vi "CPP-Multiplot.vi"(0 "Plot Array":cluster{dbl[], dbl[]}[](array[cluster]) {"?" format="%.2f"; "?" format="%.2f"}, 1 "Job Directory":path) -> (2 "Saved Automatically?":bool, 3 "gnuplotScript":string, 4 "Plot data file":path)   [LabVIEW 2012]
uses:
  gnuplotScriptComponents/plotstyle.ctl
  gnuplotScriptComponents/graphPeripherals.ctl
  gnuplotScriptComponents/minAndMax.ctl
  gnuplotScriptComponents/AxisScale.ctl
  gnuplotScriptComponents/ticsAndGrids.ctl
  gnuplotScriptComponents/tics.ctl
  gnuplotScriptComponents/grids.ctl
  gnuplotScriptComponents/legendProperties.ctl
  gnuplotScriptComponents/legendAppearance.ctl
  gnuplotScriptComponents/alignment.ctl
  gnuplotScriptComponents/at.ctl
  gnuplotScriptComponents/margins.ctl
  gnuplotScriptComponents/source.ctl
  gnuplotScriptComponents/axisName.ctl
  Results_plotter_Global.vi
panel:
  in  "OpenLogfile?":bool
  in  "Show Script Editor?":bool
  in  "Tab Control":T1(tab)
  in  "ManualPlotTitles":string[](array[string])=["", "", "", "", "", "", "", "", "", "", "", "", "", "", "", ""]
  out "AutoPlotTitles":string[](array[string])
  in  "Individual Plot Titles":bool=TRUE
  in  "Page Title Pre Block":string
  in  "Page Title Post Block":string
  in  "Values to include in Page Title":i32[](listbox)
  in  "Plotstyles":T2[](array[typedef])=[{"Style"="linespoints", "Color"=16711680, "PointType"=1, "PointSize"=1.0000001, "LineWidth"=1.0, "LineType"=1}, {"Style"="linespoints", "Color"=16860, "PointType"=2, "PointSize"=1.0000001, "LineWidth"=1.0, "LineType"=1}, {"Style"="linespoints", "Color"=51228, "PointType"=3, "PointSize"=1.0, "LineWidth"=1.0, "LineType"=1}, {"Style"="linespoints", "Color"=0, "PointType"=4, "PointSize"=1.0, "LineWidth"=1.0, "LineType"=1}] caption="Style                      Colour    PointType       PointSize         Linewidth        Linestyle" {"LineType" min=1 max=6 step=1; "LineWidth" min=1 max=6 step=1; "PointSize" min=0 step=0.1}
  out "No of Graph Slots Available":i32
  out "No of Series supplied":i32
  in  "Title Offset (characters)":cluster{"horizontal":dbl, "vertical":dbl}
  in  "Each Graph contains:":T3=enum."Series"
  in  "Rows from:":T3=enum."Until done"
  in  "Columns from:":T3=enum."Selector 1"
  in  "Margins":T4={"Top"=2.0, "Bottom"=2.0, "Left"=2.0, "Right"=2.0}
  in  "Height (in)":dbl=7.0 min=0.5 step=0.5 format="%.1f"
  in  "Width (in)":dbl=10.0 min=0.5 step=0.5 format="%.1f"
  in  "nRows":u8=3 min=1
  in  "nCols":u8=3 min=1
  in  "ScaleAdjust":dbl=0.9 min=0.1 max=2.0 step=0.1
  in  "X axis label":enum32{"Autolabel", "Manual Label"}(tab)
  out "X or theta label":string
  in  "X or theta label Manual":string
  in  "LegendProperties":T5={"Appearance"={"layout"="", "text-sample order"="", "key order"="", "surroundingBox"=""}, "Alignment"={"Horizontal"="", "Vertical"=""}, "Location"="auto", "\"At\" location"={"XcoordSys"="", "YcoordSys"="", "Xvalue"=0.0, "Yvalue"=0.0}}
  in  "Y/R tics And Grids":T9={"tics"={"Auto"=TRUE, "ticMin"=-10.0, "ticStep"=1.0, "ticMax"=10.0, "minorDivsPerMajor"=2, "Mirror tics"=TRUE}, "Grids"={"Gridlines"=enum."Major grid", "Zeroaxis"=enum."No zero axis"}}
  in  "X/Theta tics And Grids":T9={"tics"={"Auto"=TRUE, "ticMin"=-10.0, "ticStep"=1.0, "ticMax"=10.0, "minorDivsPerMajor"=2, "Mirror tics"=TRUE}, "Grids"={"Gridlines"=enum."Major grid", "Zeroaxis"=enum."No zero axis"}}
  in  "PlotType":enum32{"XY", "Polar"}(tab)
  in  "yAxisBounds":T12={"Min"={"Auto"=TRUE, "Value"=0.0}, "Max"={"Auto"=TRUE, "Value"=0.0}}
  in  "Additional XYgnuplot":string
  in  "xAxisBounds":T12={"Min"={"Auto"=TRUE, "Value"=0.0}, "Max"={"Auto"=TRUE, "Value"=0.0}}
  in  "Angle Units":bool=TRUE
  in  "AngleMode":string(combo)="Compass"
  in  "wrapGapsUpTo:":dbl=30.0 step=0.1
  in  "Additional Polar gnuplot":string
  in  "rAxisBounds":T12={"Min"={"Auto"=FALSE, "Value"=0.0}, "Max"={"Auto"=FALSE, "Value"=1.5}}
  in  "Y axis label":enum32{"Autolabel", "Manual Label"}(tab)
  out "Y or R label":string
  in  "Y or R label Manual 2":string
  in  "Edge Axis Labels only":bool=TRUE
  in  "GraphPeripherals":T14[][](array[typedef])
  out "PlotCommand":string
  in  "Filename Max length":i32=255
  out "Path":path
  out "Final Title":string
  out "AuditTrail":string[](array[string])
  out "Plot Legends":string[](array[string])
  out "Desired Legends":string[][](array[string])
  # "Overall Page Title"
  # "Plot Styles"
  # "There are as many graphs as there are titles (from Selector 2)...."
  # "And each graph contains plots from Selector 1..."
  # "Rows/ Columns/ Series from: controls not wired- just a thought for explicit control of what goes where...?"
  # "X/theta"
  # "Y/r"
  # "Shows the numbered line colours and point styles available"
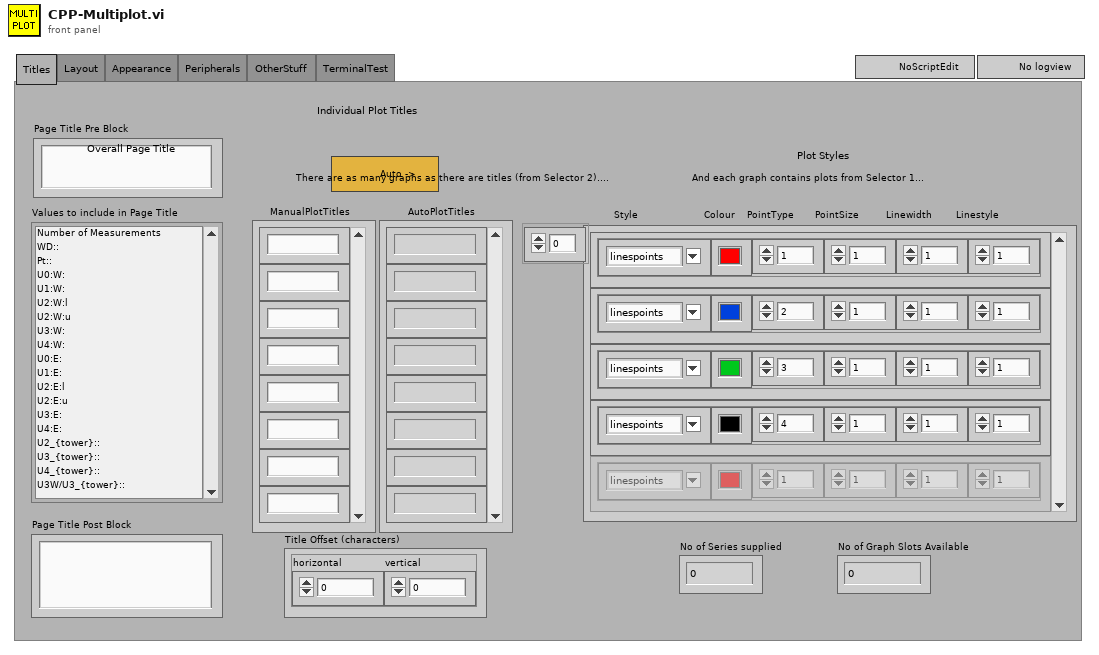
[diagram p1: front panel]
types:
  T1 = enum32{"Titles", "Layout", "Appearance", "Peripherals", "OtherStuff ", "TerminalTest"}
  T2 = typedef "plotstyle.ctl" = cluster{"Style":string, "Color":u32, "PointType":i32, "PointSize":sgl, "LineWidth":sgl, "LineType":u8}
  T3 = typedef "source.ctl" = enum16{"Specified:", "Selector 1", "Selector 2", "Until done", "Series"}
  T4 = typedef "margins.ctl" = cluster{"Top":dbl, "Bottom":dbl, "Left":dbl, "Right":dbl}
  T5 = typedef "legendProperties.ctl" = cluster{"Appearance":T6, "Alignment":T7, "Location":string, "\"At\" location":T8}
  T6 = typedef "legendAppearance.ctl" = cluster{"layout":string, "text-sample order":string, "key order":string, "surroundingBox":string}
  T7 = typedef "alignment.ctl" = cluster{"Horizontal":string, "Vertical":string}
  T8 = typedef "at.ctl" = cluster{"XcoordSys":string, "YcoordSys":string, "Xvalue":dbl, "Yvalue":dbl}
  T9 = typedef "ticsAndGrids.ctl" = cluster{"tics":T10, "Grids":T11}
  T10 = typedef "tics.ctl" = cluster{"Auto":bool, "ticMin":dbl, "ticStep":dbl, "ticMax":dbl, "minorDivsPerMajor":i32, "Mirror tics":bool}
  T11 = typedef "grids.ctl" = cluster{"Gridlines":enum16{"No grids", "Major grid", "Minor grid", "Major and Minor"}, "Zeroaxis":enum16{"No zero axis", "Show zero axis"}}
  T12 = typedef "minAndMax.ctl" = cluster{"Min":T13, "Max":T13}
  T13 = typedef "AxisScale.ctl" = cluster{"Auto":bool, "Value":dbl}
  T14 = typedef "graphPeripherals.ctl" = cluster{"title":bool, "key":bool, "Xtic":bool, "Ytic":bool, "Xlab":bool, "Ylab":bool}
  T15 = typedef "axisName.ctl" = string
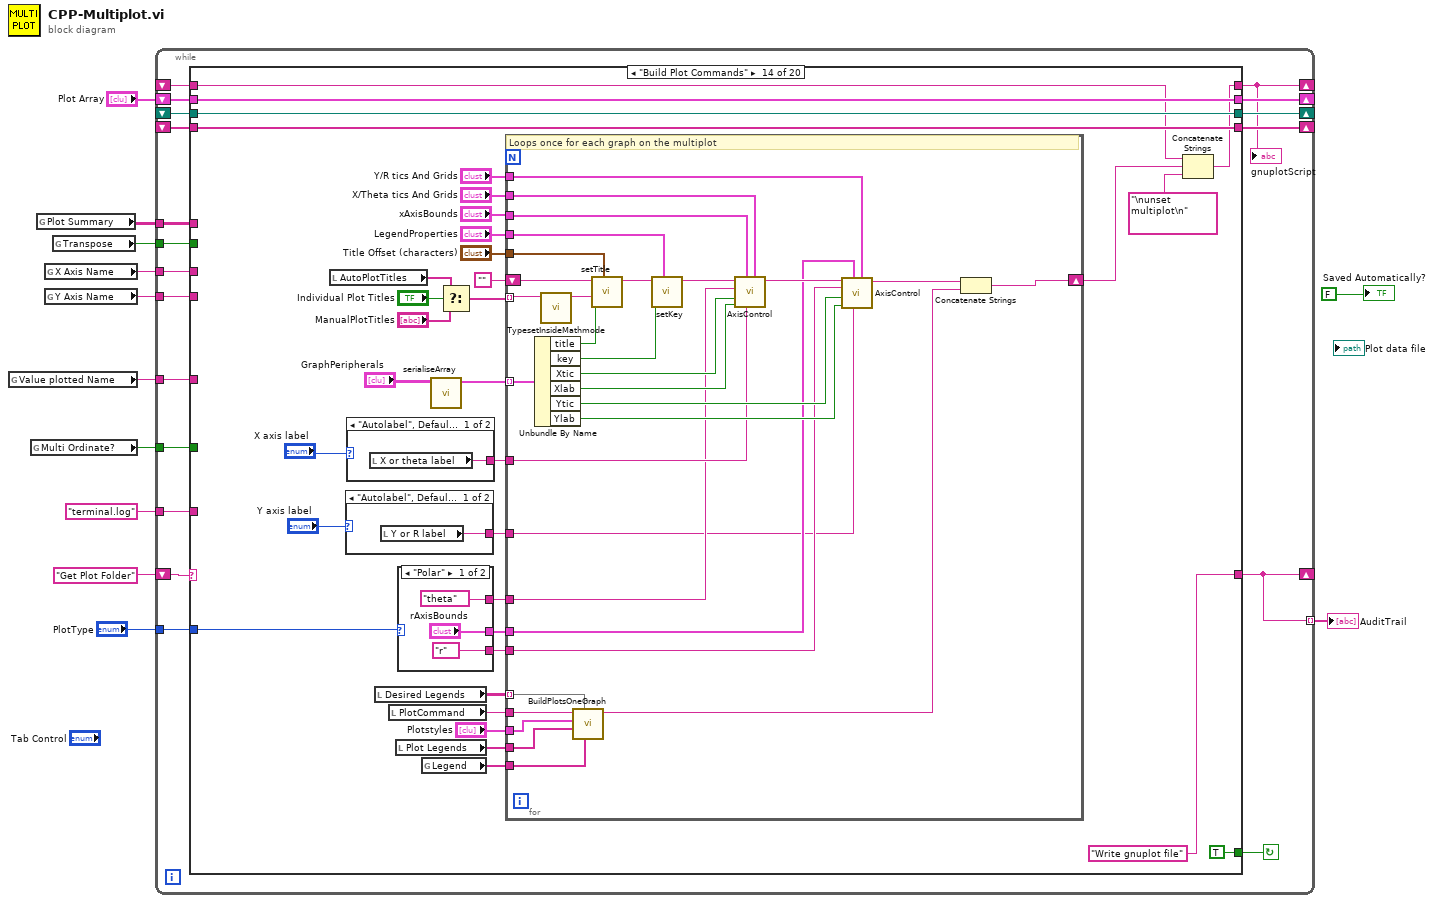
[diagram p0: block diagram]
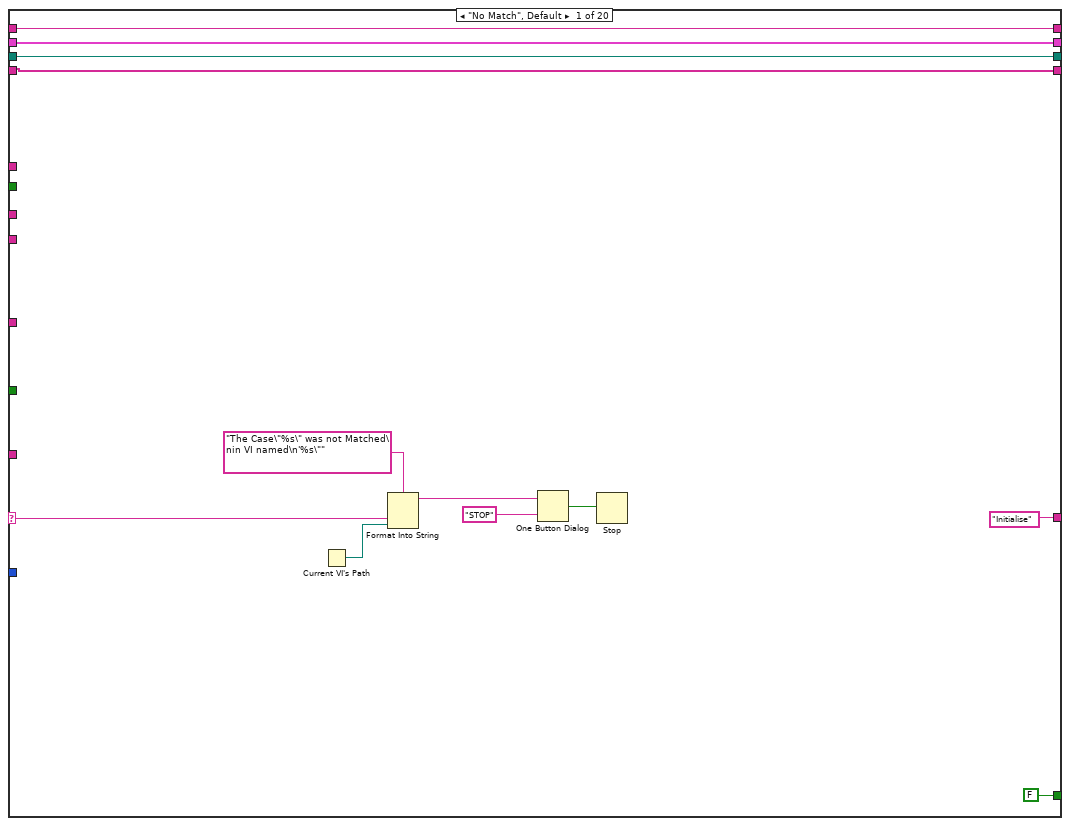
[diagram p2: hidden frame]
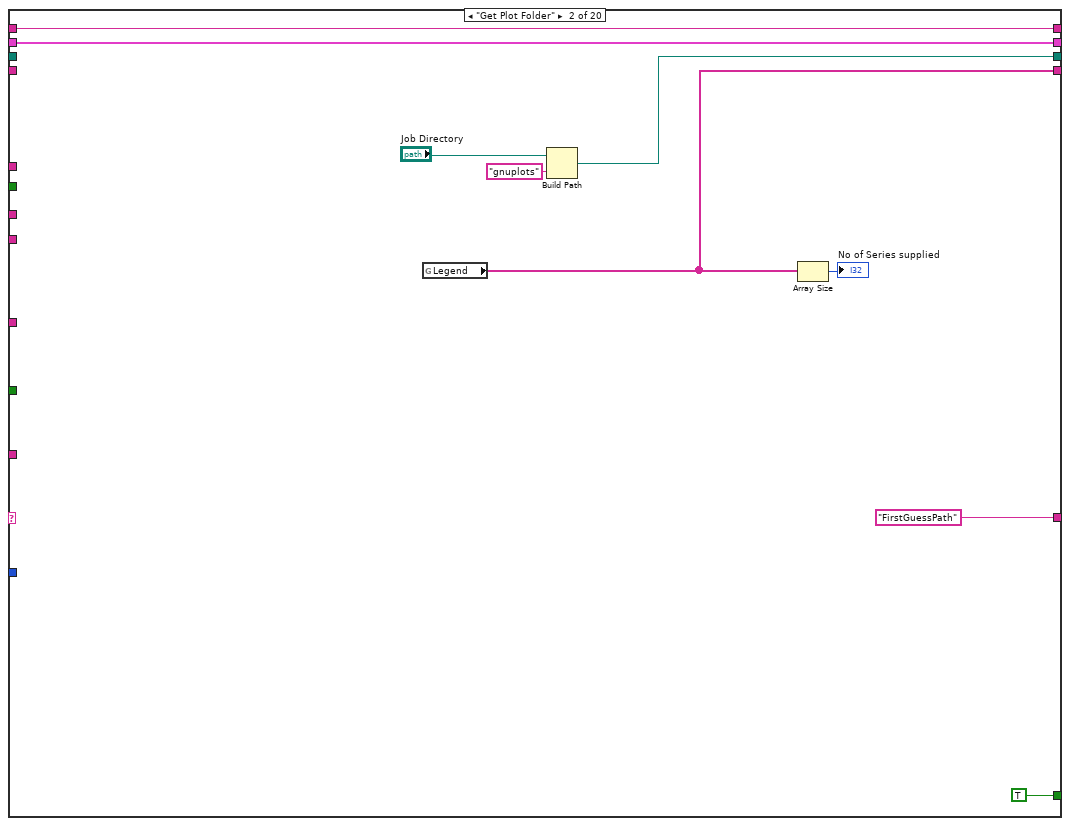
[diagram p3: hidden frame]
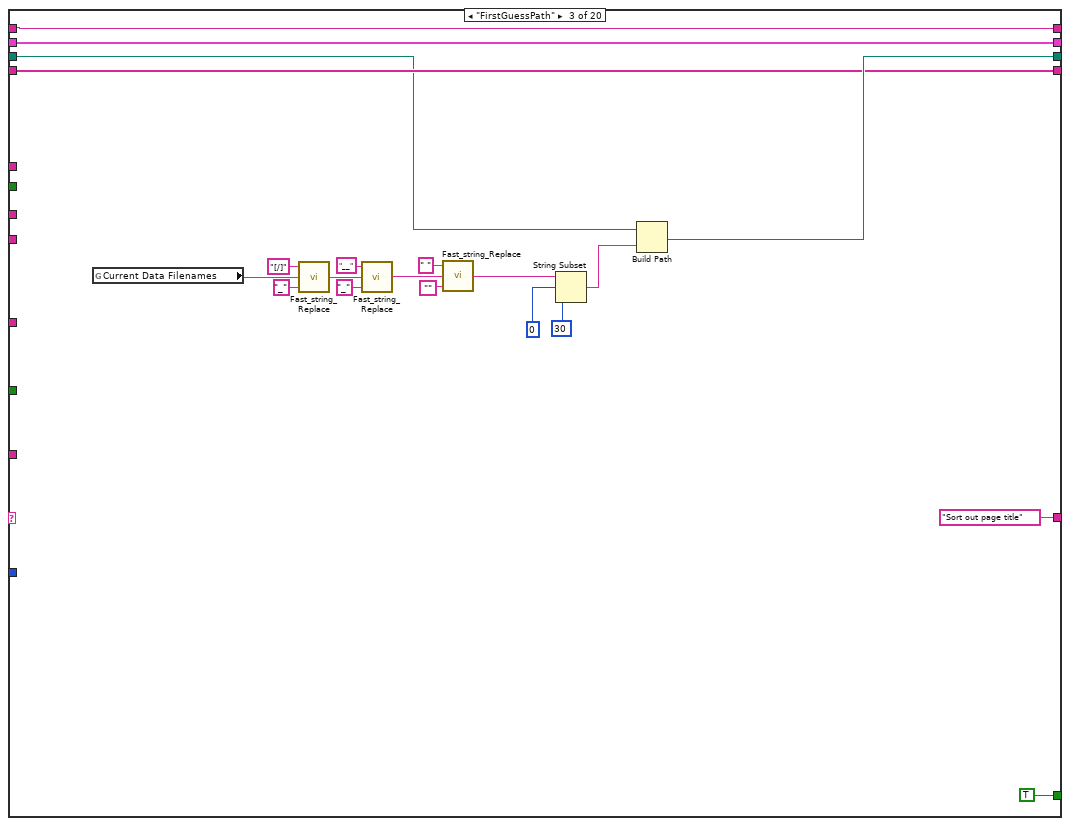
[diagram p4: hidden frame]
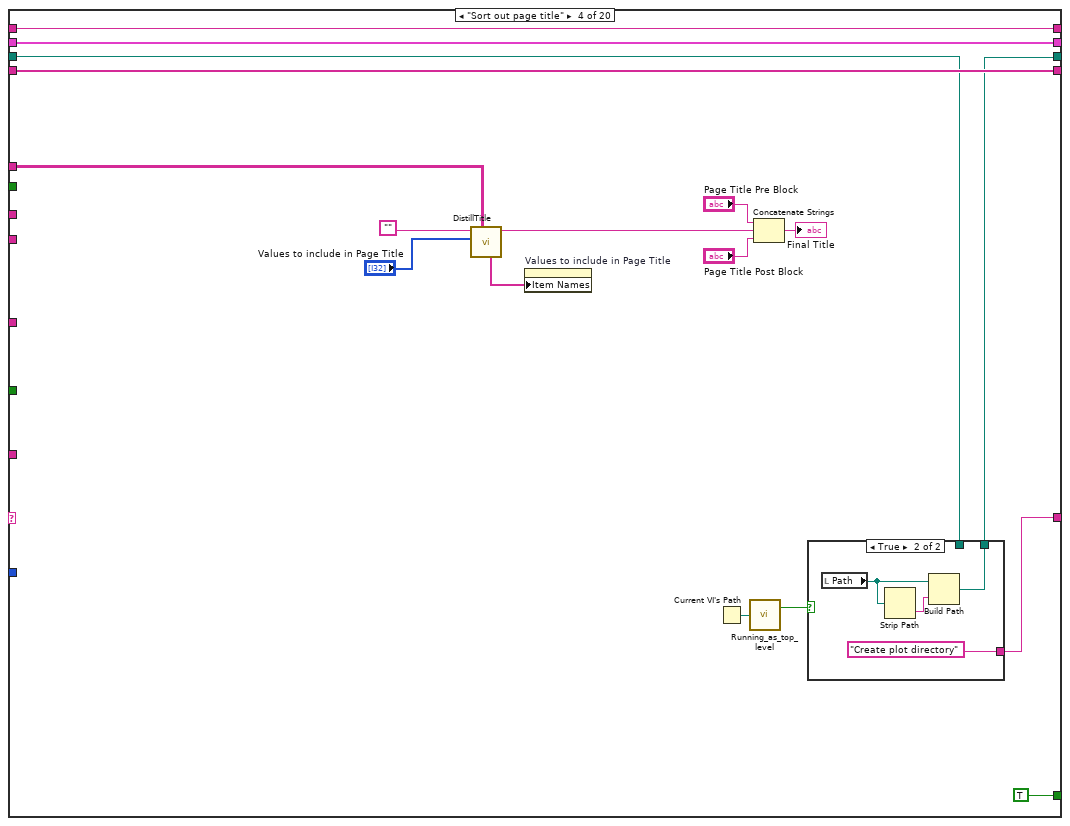
[diagram p5: hidden frame]
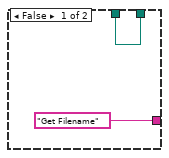
[diagram p6: hidden frame]
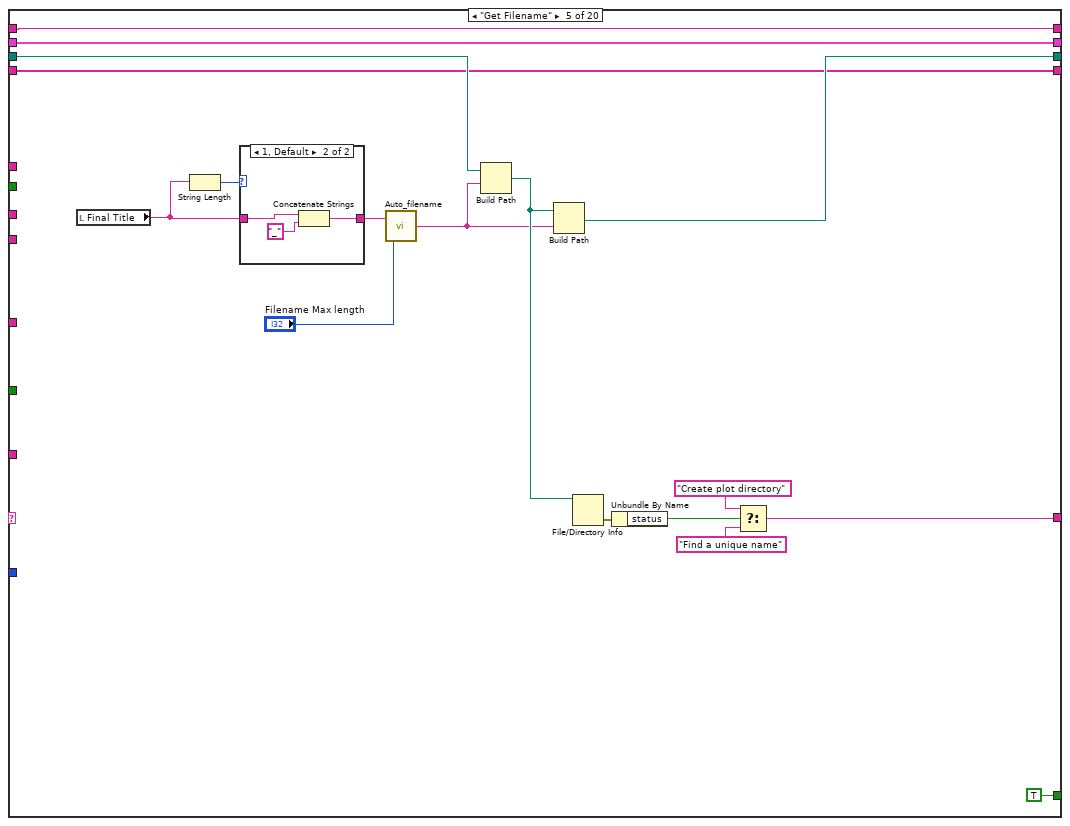
[diagram p7: hidden frame]
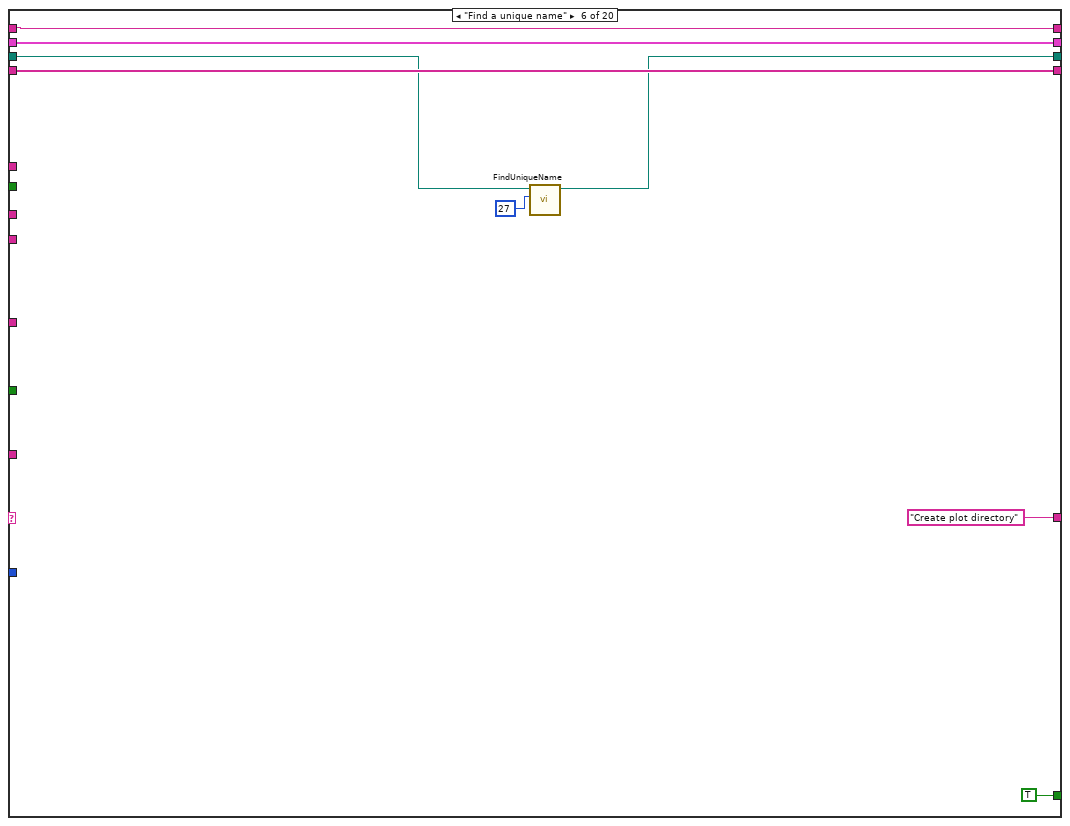
[diagram p9: hidden frame]
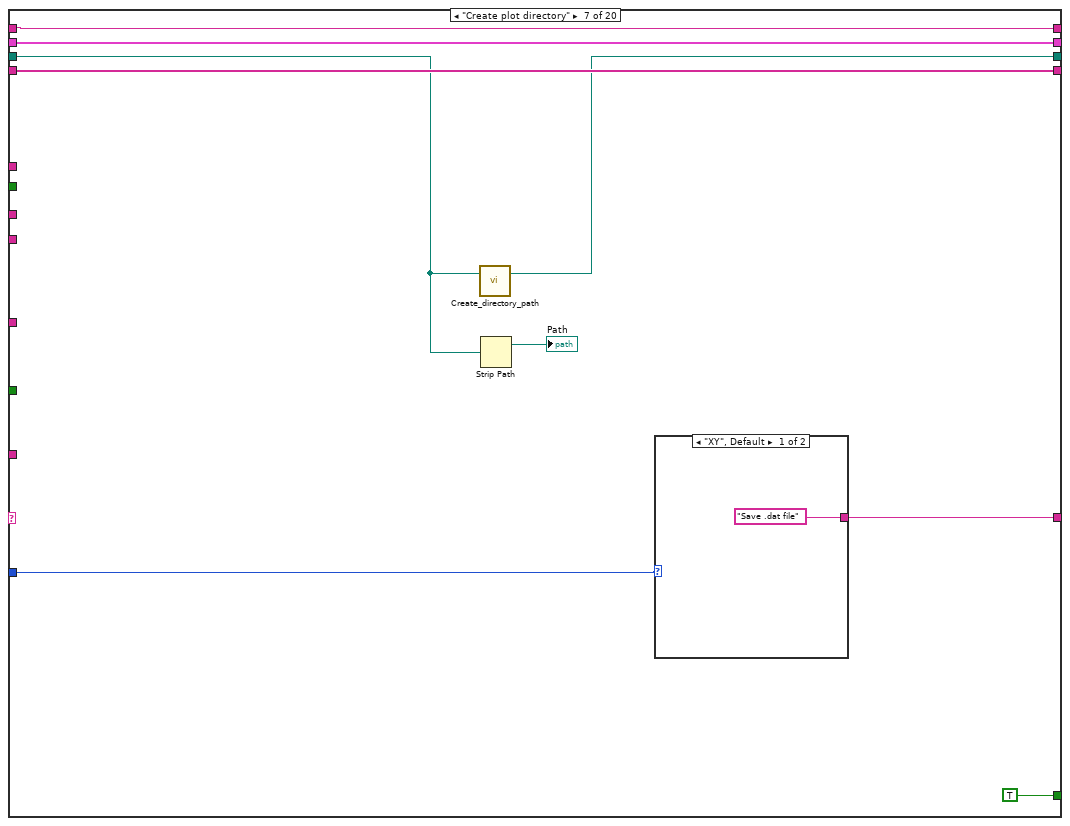
[diagram p10: hidden frame]
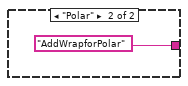
[diagram p11: hidden frame]
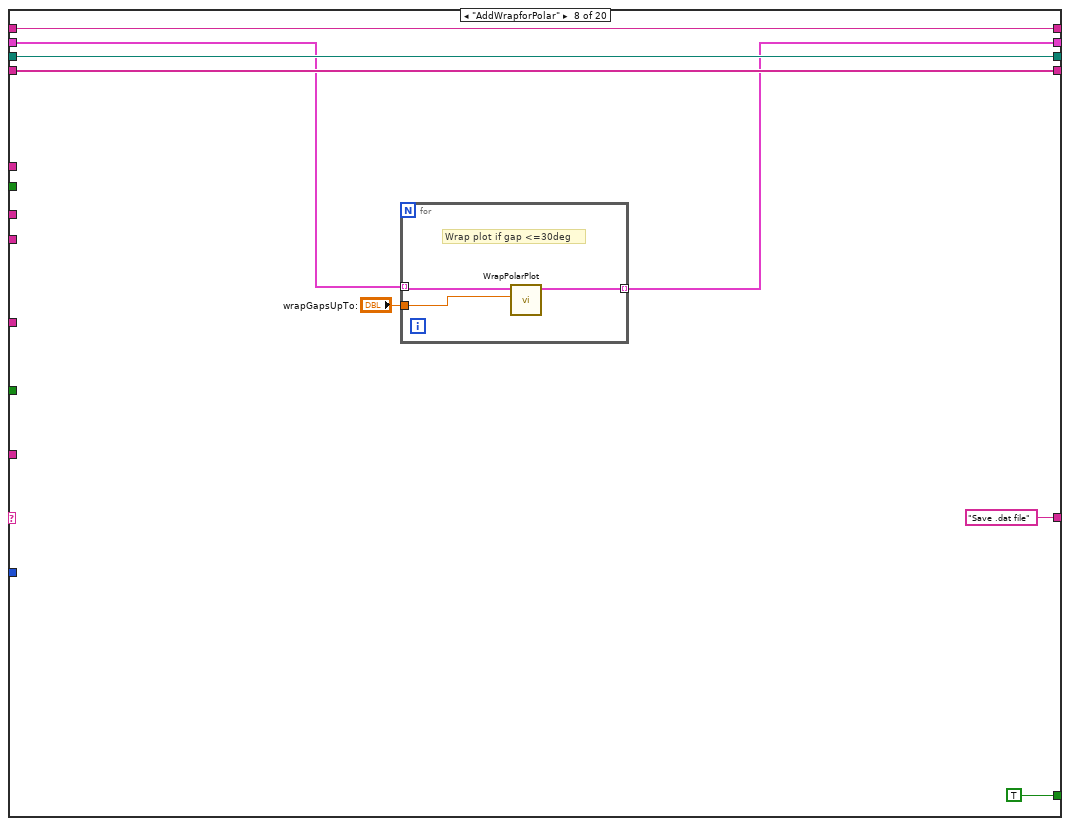
[diagram p12: hidden frame]
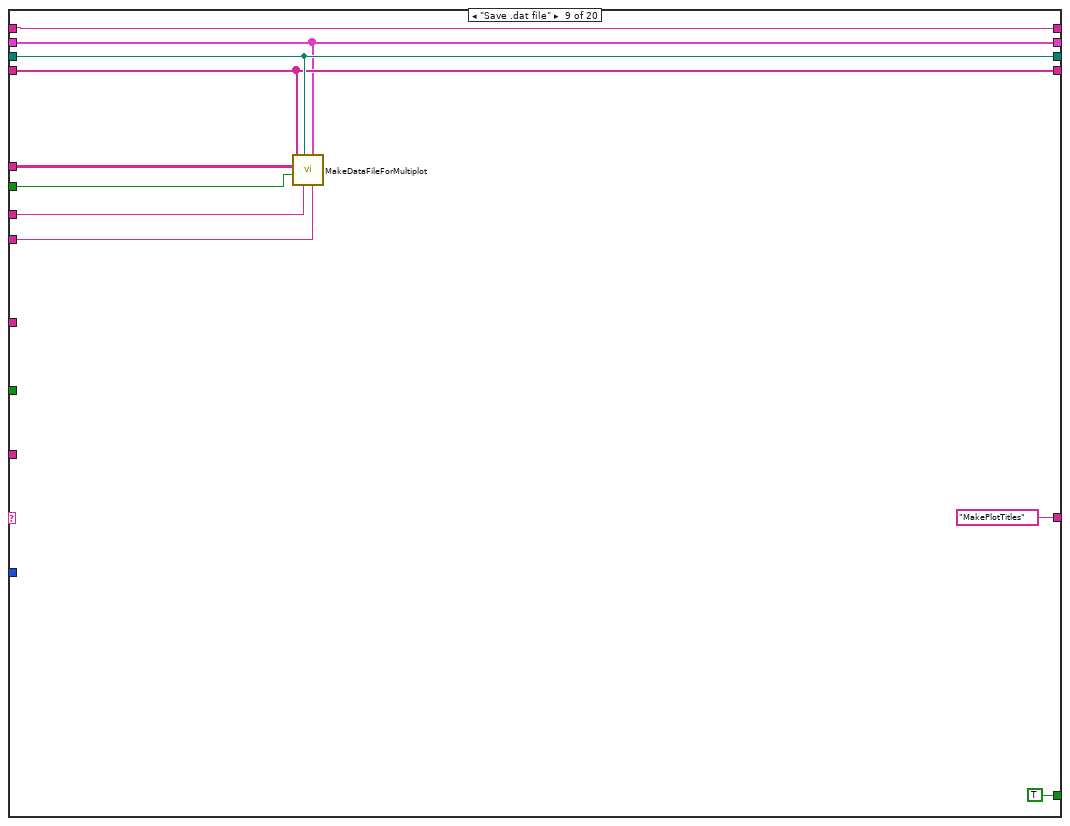
[diagram p13: hidden frame]
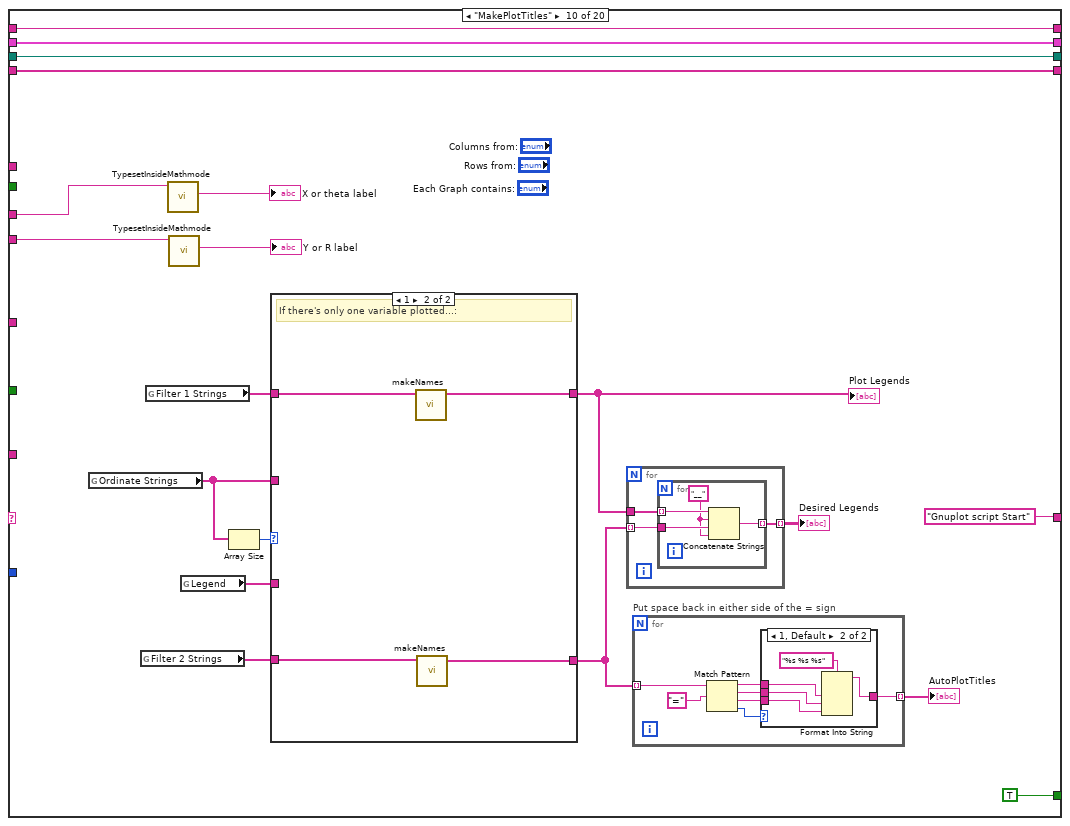
[diagram p14: hidden frame]
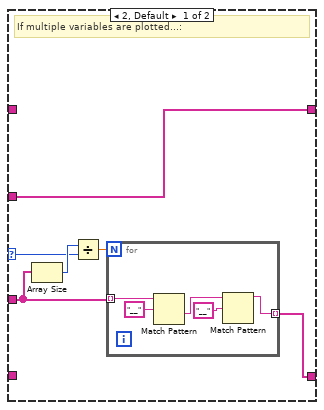
[diagram p16: hidden frame]
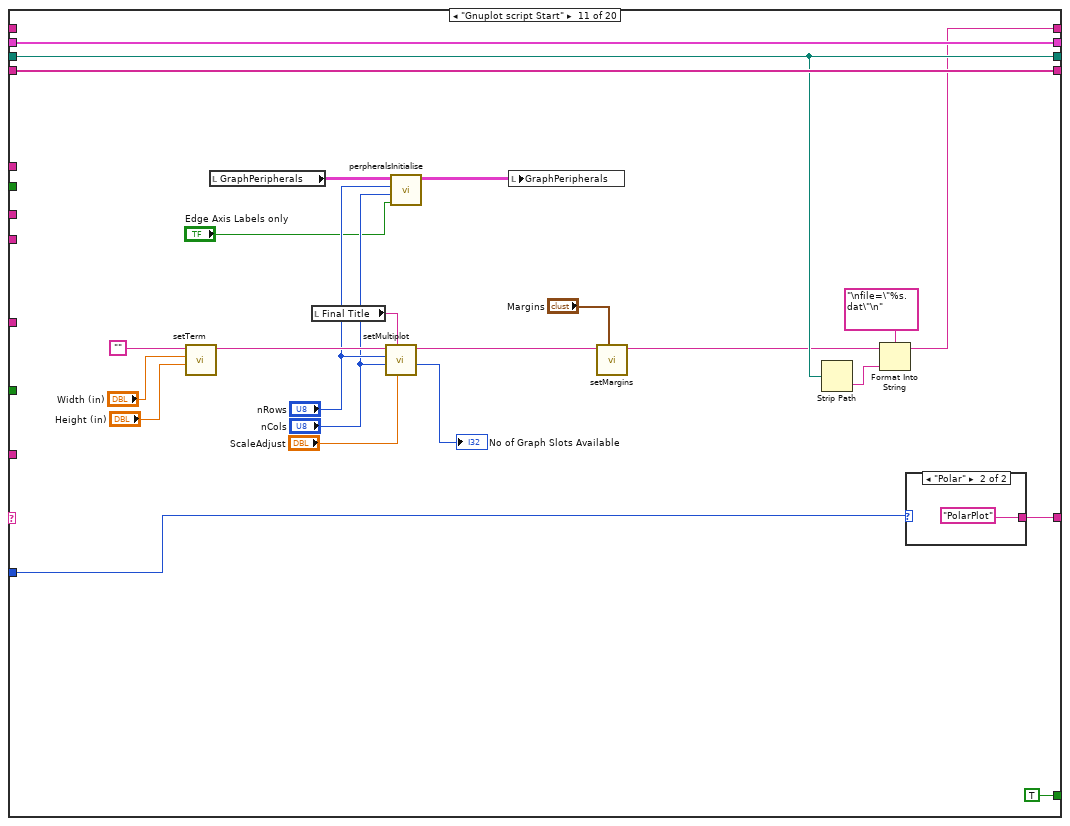
[diagram p17: hidden frame]
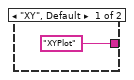
[diagram p18: hidden frame]
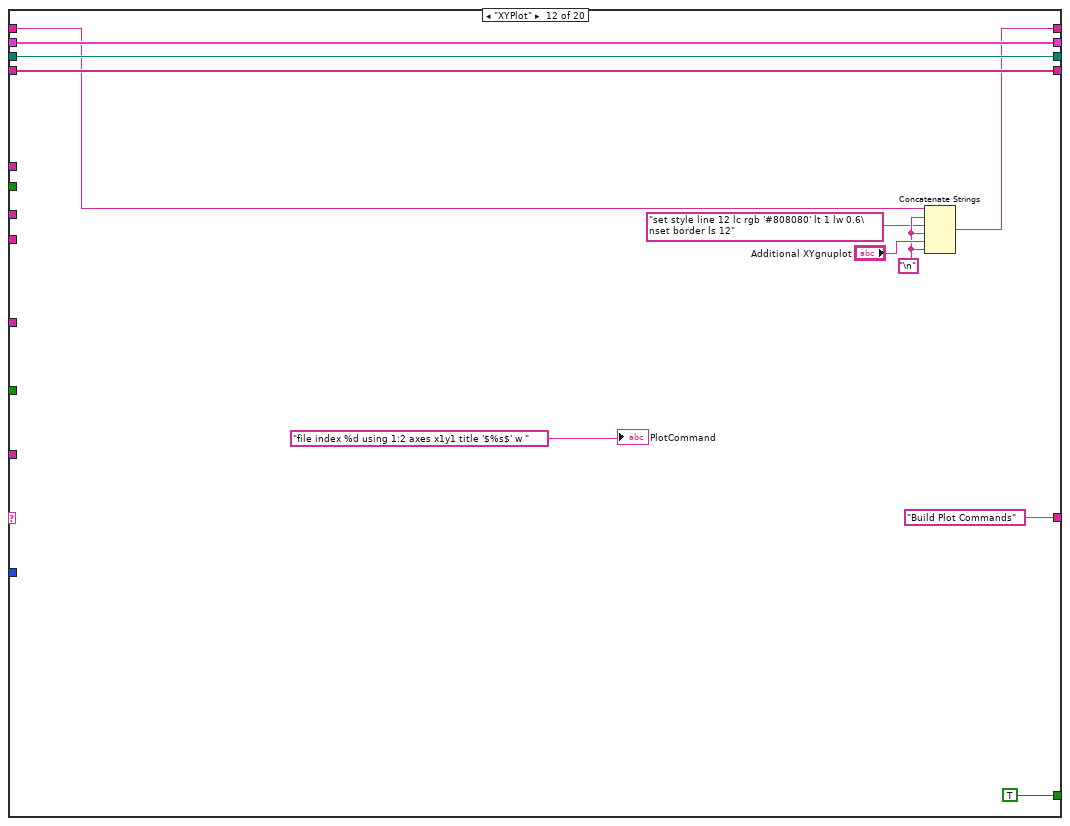
[diagram p19: hidden frame]
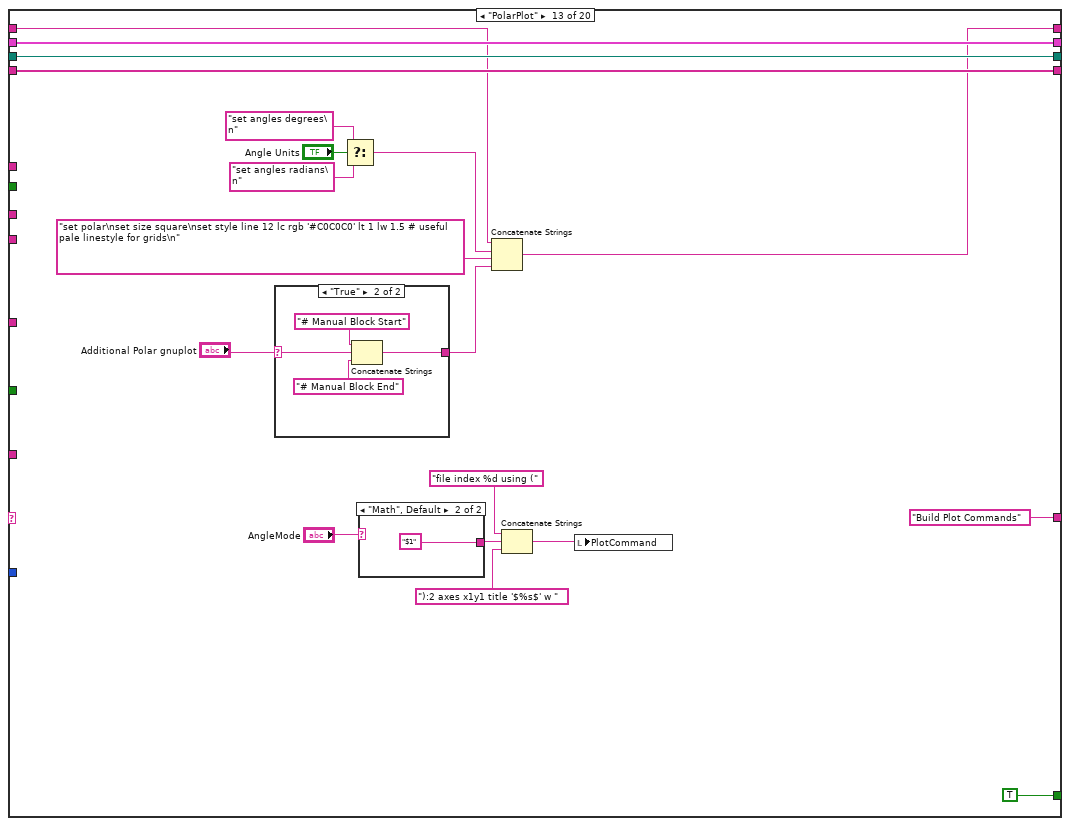
[diagram p20: hidden frame]
diagram:
  n1 = global read "Results_plotter_Global.vi" "Value plotted Name"() -> (w8:string)
  n2 = global read "Results_plotter_Global.vi" "Multi Ordinate?"() -> (w3:bool)
  n3 = global read "Results_plotter_Global.vi" "Plot Summary"() -> (w11:string[][])
  n4 = global read "Results_plotter_Global.vi" "X Axis Name"() -> (w10:string)
  n5 = global read "Results_plotter_Global.vi" "Y Axis Name"() -> (w9:string)
  n6 = global read "Results_plotter_Global.vi" "Transpose"() -> (w4:bool)
  n7 = while {
    shift-left: "Get Plot Folder" -> [w30]
    shift-right: [w14] -> _
    tunnel: w11 -> [w29]
    shift-right: [w28] -> _
    shift-left: _ -> [w27]
    tunnel: w10 -> [w26]
    tunnel: w9 -> [w25]
    tunnel: w8 -> [w24]
    shift-right: [w22] -> _
    shift-left: "Plot Array" -> [w23]
    shift-right: [w15] -> _
    shift-left: _ -> [w21]
    shift-right: [w20] -> _
    shift-left: _ -> [w19]
    tunnel: "terminal.log" -> [w18]
    tunnel: w4 -> [w17]
    tunnel: w3 -> [w16]
    tunnel: [w14] -> w2 mode=indexing
    tunnel: "PlotType" -> [w13]
    stop <- w31 continue-if-true
    n8 = case shown="\"Build Plot Commands\"" w30 {
      selector: w30 -> [w32 _ _ _ _ _ _ _ _ _ _ _ _ _ _ _ _ _ _ _]
      tunnel: [FALSE TRUE TRUE ("Top Level") TRUE ("Top Level") TRUE ("Top Level") TRUE ("Top Level") TRUE TRUE ("Top Level") TRUE ("Top Level") TRUE ("Top Level") TRUE ("Top Level") TRUE ("Top Level") TRUE ("Top Level") TRUE ("Top Level") TRUE ("Top Level") TRUE ("Top Level") TRUE ("Top Level") FALSE ("Top Level") TRUE ("Top Level") FALSE ("Top Level")] -> w31
      tunnel: ["Initialise" "FirstGuessPath" "Sort out page title" w81 w110 "Create plot directory" w125 "Save .dat file" "MakePlotTitles" "Gnuplot script Start" w231 "Build Plot Commands" "Build Plot Commands" "Write gnuplot file" ("t") "Execute shell script" ("t") "Has pdf been generated?" ("t") w371 "End" "End" ("t") "End" ("t")] -> w14
      tunnel: w29 -> [_ _ _ w75 _ _ _ _ w154 _ _ _ _ _ _ _ _ _ _ _]
      tunnel: [w36 w50 w72 w83 w111 w117 w130 w142 w155 w175 w222 w247 w265 w306 w353 w361 w375 w380 w390 w401] -> w28
      tunnel: w27 -> [w36 _ w68 w82 w107 w118 w129 w142 w155 w175 w222 w247 w265 w306 w353 w361 w375 w380 w390 w401]
      tunnel: w26 -> [_ _ _ _ _ _ _ _ w153 w168 _ _ _ _ _ _ _ _ _ _]
      tunnel: w25 -> [_ _ _ _ _ _ _ _ w152 w167 _ _ _ _ _ _ _ _ _ _]
      tunnel: w24 -> [_ _ _ _ _ _ _ _ _ _ _ _ _ _ _ _ _ _ _ _]
      tunnel: w23 -> [w35 w46 w71 w89 w109 w121 w133 w138 w149 w174 w234 w246 w266 w307 w359 w366 w378 w385 w395 w400]
      tunnel: [w35 w46 w71 w89 w109 w121 w133 w137 w149 w174 w234 w246 w266 w307 w359 w366 w378 w385 w395 w400] -> w22
      tunnel: w21 -> [w34 w49 w70 w87 w108 w120 w132 w143 w156 w173 _ w237 w260 w298 w349 w364 w376 w383 w393 w399]
      tunnel: [w34 w49 w70 w87 w108 w120 w132 w143 w156 w173 w219 w241 w261 w304 w349 w364 w376 w383 w393 w399] -> w15
      tunnel: [w33 w45 w69 w88 w106 w119 w131 w141 w151 w172 w233 w245 w264 w305 w354 w365 w377 w384 w394 w398] -> w20
      tunnel: w19 -> [w33 _ w69 w88 w106 w119 w131 w141 w151 w172 w233 w245 w264 w305 w354 w365 w377 w384 w394 w398]
      tunnel: w18 -> [_ _ _ _ _ _ _ _ _ _ _ _ _ _ _ w360 _ _ w388 _]
      tunnel: w17 -> [_ _ _ _ _ _ _ _ w150 _ _ _ _ _ _ _ _ _ _ _]
      tunnel: w16 -> [_ _ _ _ _ _ _ _ _ _ _ _ _ _ _ _ _ _ _ _]
      tunnel: w13 -> [_ _ _ _ _ _ w126 _ _ _ w218 _ _ w282 _ _ _ _ _ _]
      frame "No Match", Default {
        n9 = Current VI's Path() -> (path=w38:path)
        n10 = Format Into String(format string="The Case\"%s\" was not Matched\nin VI named\n'%s\"" ("Format String"), w32, w38) -> (resulting string=w41:string)  [unwired: 2 in, 1 out]
        n11 = One Button Dialog(message=w41, button name ("OK")="STOP") -> (true=w39:bool)
        n12 = Stop(stop? (T)=w39) -> ()
      }
      frame "Get Plot Folder" {
        n13 = global read "Results_plotter_Global.vi" "Legend"() -> (w45:string[])
        n14 = Build Path(base path="Job Directory", name or relative path="gnuplots") -> (appended path=w50:path)
        n15 = Array Size(array=w45) -> (size(s)=→"No of Series supplied":i32)
      }
      frame "FirstGuessPath" {
        n16 = global read "Results_plotter_Global.vi" "Current Data Filenames"() -> (w57:string)
        n17 = call "Fast_string_Replace.vi"("Replace match with:"="_", "Input String"=w57, "regular expression"="[/]") -> ("Output String"=w61:string)  [unwired: 2 out]
        n18 = call "Fast_string_Replace.vi"("Replace match with:"="_", "Input String"=w61, "regular expression"="__") -> ("Output String"=w58:string)  [unwired: 2 out]
        n19 = call "Fast_string_Replace.vi"("Replace match with:"="", "Input String"=w58, "regular expression"=" ") -> ("Output String"=w56:string)  [unwired: 2 out]
        n20 = String Subset(string=w56, offset (0)=0, length (rest)=30 ("length (rest)")) -> (substring=w55:string)
        n21 = Build Path(base path=w68, name or relative path=w55) -> (appended path=w72:path)
      }
      frame "Sort out page title" {
        n22 = call "DistillTitle.vi"("Plot Summary in"=w75, "Indices to include in Page Title"="Values to include in Page Title", "String in"="") -> ("String out"=w80:string, "AvailableVariables"=w73:string[])  [unwired: 7 in]
        n23 = property on="Values to include in Page Title" class="LstBox (strict)"("Item Names"=w73) -> ()  [unwired: 2 in, 2 out]
        n24 = Current VI's Path() -> (path=w86:path)
        n25 = call "Running_as_top_level.vi"("Vi path name"=w86) -> ("Top Level"=w84:bool)  [unwired: 1 out]
        n26 = Concatenate Strings("Page Title Pre Block", w80, "Page Title Post Block") -> (→"Final Title":string)
        n27 = case shown="True" w84 {
          tunnel: [w91 w94] -> w83
          tunnel: w82 -> [w91 _]
          tunnel: ["Get Filename" ("t") "Create plot directory"] -> w81
          frame False {
          }
          frame True {
            n28 = local read "Path"() -> (w93:path)
            n29 = Strip Path(path=w93) -> (name=w92:string)  [unwired: 1 out]
            n30 = Build Path(base path=w93, name or relative path=w92) -> (appended path=w94:path)
          }
        }
      }
      frame "Get Filename" {
        n31 = local read "Final Title"() -> (w96:string)
        n32 = String Length(string=w96) -> (length=w98:i32)
        n33 = case shown="1, Default" w98 {
          tunnel: [w113 w114] -> w97
          tunnel: w96 -> [w113 w116]
          frame 0 {
          }
          frame 1, Default {
            n34 = Concatenate Strings(w116, "_") -> (w114:string)
          }
        }
        n35 = call "Auto_filename.vi"("Filename Max length"="Filename Max length", "Prefix"=w97) -> ("Filename"=w100:string)
        n36 = Build Path(base path=w107, name or relative path=w100) -> (appended path=w104:path)
        n37 = Build Path(base path=w104, name or relative path=w100) -> (appended path=w111:path)
        n38 = File/Directory Info(path=w104) -> (error out=w105:errorcluster)  [unwired: 1 in, 6 out]
        n39 = Unbundle By Name(w105) -> ("status"=w103:bool)
        n40 = Select(t="Create plot directory", s=w103, f="Find a unique name") -> (s? t:f=w110:string)
      }
      frame "Find a unique name" {
        n41 = call "FindUniqueName.vi"("Max Length"=27, "PathIn"=w118) -> ("UniquedPath"=w117:path)  [unwired: 9 in]
      }
      frame "Create plot directory" {
        n42 = call "Create_directory_path.vi"("Path name"=w129) -> ("Path name Out"=w130:path)  [unwired: 1 in, 1 out]
        n43 = Strip Path(path=w129) -> (stripped path=→"Path":path)  [unwired: 1 out]
        n44 = case shown="\"XY\", Default" w126 {
          tunnel: ["Save .dat file" "AddWrapforPolar"] -> w125
          frame "XY", Default {
          }
          frame "Polar" {
          }
        }
      }
      frame "AddWrapforPolar" {
        n45 = for {
          tunnel: w138 -> [w146] mode=indexing
          tunnel: [w145] -> w137 mode=indexing
          tunnel: "wrapGapsUpTo:" -> [w144]
          # "Wrap plot if gap <=30deg"
          n46 = call "WrapPolarPlot.vi"("maxWrap"=w144, "thetaRin"=w146) -> ("thetaRout"=w145:cluster{"Angle":dbl[], "Radius":dbl[]})  [unwired: 9 in]
        }
      }
      frame "Save .dat file" {
        n47 = call "MakeDataFileForMultiplot.vi"("Y Axis Name"=w152, "Plot Array"=w149, "X Axis Name"=w153, "Path"=w155, "Transpose"=w150, "Plot Summary"=w154, "Legend"=w151) -> ()  [unwired: 5 in]
      }
      frame "MakePlotTitles" {
        n48 = global read "Results_plotter_Global.vi" "Ordinate Strings"() -> (w166:string[])
        n49 = global read "Results_plotter_Global.vi" "Filter 2 Strings"() -> (w163:string[])
        n50 = global read "Results_plotter_Global.vi" "Filter 1 Strings"() -> (w164:string[])
        n51 = call "TypesetInsideMathmode.vi"("DirtyString"=w168) -> ("Mathmode String"=→"X or theta label":string)  [unwired: 9 in, 1 out]
        n52 = call "TypesetInsideMathmode.vi"("DirtyString"=w167) -> ("Mathmode String"=→"Y or R label":string)  [unwired: 9 in, 1 out]
        n53 = global read "Results_plotter_Global.vi" "Legend"() -> (w170:string[])
        n54 = Array Size(array=w166) -> (size(s)=w159:i32)
        n55 = case shown="1" w159 {
          selector: w159 -> [w196 _]
          tunnel: w170 -> [w199 _]
          tunnel: [w201 w208] -> w162
          tunnel: [w200 w210] -> w160
          tunnel: w166 -> [w200 _]
          tunnel: w164 -> [_ w209]
          tunnel: w163 -> [_ w207]
          frame 2, Default {
            # "If multiple variables are plotted...:"
            n56 = Array Size(array=w199) -> (size(s)=w198:i32)
            n57 = Divide(x=w198, y=w196) -> (x/y=w197:dbl)
            n58 = for {
              N: w197 -> [_]
              tunnel: w199 -> [w205] mode=indexing
              tunnel: [w202] -> w201 mode=indexing
              n59 = Match Pattern(string=w205, regular expression="__") -> (after substring=w203:string)  [unwired: 1 in, 3 out]
              n60 = Match Pattern(string=w203, regular expression="__") -> (before substring=w202:string)  [unwired: 1 in, 3 out]
            }
          }
          frame 1 {
            # "If there's only one variable plotted...:"
            n61 = call "makeNames.vi"("Strings"=w209) -> ("Names"=w210:string[])  [unwired: 10 in]
            n62 = call "makeNames.vi"("Strings"=w207) -> ("Names"=w208:string[])  [unwired: 10 in]
          }
        }
        "Plot Legends" <- w160
        n63 = for {
          tunnel: w160 -> [w191]
          tunnel: w162 -> [w190] mode=indexing
          tunnel: [w189] -> w165 mode=indexing
          n64 = for {
            tunnel: w191 -> [w195] mode=indexing
            tunnel: w190 -> [w194]
            tunnel: [w193] -> w189 mode=indexing
            w192 = "__" ("string")
            n65 = Concatenate Strings(w195, w192, w194, w192) -> (w193:string)
          }
        }
        "Desired Legends" <- w165
        n66 = for "Put space back in either side of the = sign" {
          tunnel: w162 -> [w182] mode=indexing
          tunnel: [w177] -> w161 mode=indexing
          n67 = Match Pattern(string=w182, regular expression="=") -> (before substring=w180:string, match substring=w179:string, after substring=w178:string, offset past match=w176:i32)  [unwired: 1 in]
          n68 = case shown="1, Default" w176 {
            tunnel: w180 -> [w183 w188]
            tunnel: w179 -> [_ w187]
            tunnel: w178 -> [_ w186]
            tunnel: [w183 w185] -> w177
            frame -1 {
            }
            frame 1, Default {
              n69 = Format Into String(format string="%s %s %s", w188, w187, w186) -> (resulting string=w185:string)  [unwired: 2 in, 1 out]
            }
          }
        }
        "AutoPlotTitles" <- w161
      }
      frame "Gnuplot script Start" {
        n70 = call "setTerm.vi"("Height (in)"="Height (in)", "Width (in)"="Width (in)", "String in"="") -> ("String out"=w227:string)  [unwired: 7 in, 1 out]
        n71 = local read "GraphPeripherals"() -> (w213:T14[][])
        n72 = local read "Final Title"() -> (w225:string)
        n73 = call "setMultiplot.vi"("ScaleAdjust"="ScaleAdjust", "OverallTitle"=w225, "Cols"="nCols", "Rows"="nRows", "String in"=w227) -> ("nGraphs"=→"No of Graph Slots Available":i32, "String out"=w226:string)  [unwired: 4 in, 1 out]
        n74 = call "perpheralsInitialise.vi"("Edge Axis Labels only"="Edge Axis Labels only", "Cols"="nCols", "Rows"="nRows", "GraphPeripheralsIn"=w213) -> ("GraphPeripheralsOut"=w214:T14[][])  [unwired: 7 in]
        n75 = local write "GraphPeripherals"(w214) -> ()
        n76 = call "setMargins.vi"("Margins"="Margins", "String in"=w226) -> ("String out"=w217:string)  [unwired: 8 in, 1 out]
        n77 = Strip Path(path=w222) -> (name=w221:string)  [unwired: 1 out]
        n78 = Format Into String(format string="\nfile=\"%s.dat\"\n" ("string"), initial string=w217, w221) -> (resulting string=w219:string)  [unwired: 1 in, 1 out]
        n79 = case shown="\"Polar\"" w218 {
          tunnel: ["XYPlot" "PolarPlot"] -> w231
          frame "XY", Default {
          }
          frame "Polar" {
          }
        }
      }
      frame "XYPlot" {
        w240 = "\n"
        n80 = Concatenate Strings(w237, w240, "set style line 12 lc rgb '#808080' lt 1 lw 0.6\nset border ls 12" ("input 2"), w240, "Additional XYgnuplot", w240) -> (w241:string)
        "PlotCommand" <- "file index %d using 1:2 axes x1y1 title '$%s$' w " ("format string")
      }
      frame "PolarPlot" {
        n81 = case shown="\"True\"" "Additional Polar gnuplot" {
          selector: "Additional Polar gnuplot" -> [w267 w271]
          tunnel: [w267 w270] -> w248
          frame "\u0000", Default {
          }
          frame "True" {
            n82 = Concatenate Strings("# Manual Block Start" ("string"), w271, "# Manual Block End" ("string")) -> (w270:string)
          }
        }
        n83 = Select(t="set angles degrees\n", s="Angle Units", f="set angles radians\n") -> (s? t:f=w250:string)
        n84 = case shown="\"Math\", Default" "AngleMode" {
          tunnel: ["90-$1" ("format string") "$1" ("format string")] -> w255
          frame "Compass" {
          }
          frame "Math", Default {
          }
        }
        n85 = Concatenate Strings(w260, w250, "set polar\nset size square\nset style line 12 lc rgb '#C0C0C0' lt 1 lw 1.5 # useful pale linestyle for grids\n", w248) -> (w261:string)
        n86 = Concatenate Strings("file index %d using (" ("format string"), w255, "):2 axes x1y1 title '$%s$' w " ("format string")) -> (w254:string)
        n87 = local write "PlotCommand"(w254) -> ()
      }
      frame "Build Plot Commands" {
        n88 = local read "AutoPlotTitles"() -> (w296:string[])
        n89 = case shown="\"Autolabel\", Default" "Y axis label" {
          tunnel: [w308 "Y or R label Manual 2"] -> w277
          frame "Autolabel", Default {
            n90 = local read "Y or R label"() -> (w308:string)
          }
          frame "Manual Label" {
          }
        }
        n91 = case shown="\"Autolabel\", Default" "X axis label" {
          tunnel: [w316 "X or theta label Manual"] -> w283
          frame "Autolabel", Default {
            n92 = local read "X or theta label"() -> (w316:string)
          }
          frame "Manual Label" {
          }
        }
        n93 = local read "Desired Legends"() -> (w290:string[][])
        n94 = local read "PlotCommand"() -> (w285:string)
        n95 = local read "Plot Legends"() -> (w291:string[])
        n96 = case shown="\"Polar\"" w282 {
          tunnel: [T15 "theta" ("Axis") T15 "x" ("Axis")] -> w280
          tunnel: [T15 "r" ("Axis") T15 "y" ("Axis")] -> w279
          tunnel: ["rAxisBounds" "yAxisBounds"] -> w281
          frame "Polar" {
          }
          frame Default {
          }
        }
        n97 = global read "Results_plotter_Global.vi" "Legend"() -> (w289:string[])
        n98 = call "serialiseArray.vi"("GraphPeripherals"="GraphPeripherals") -> ("output array"=w292:T14[])  [unwired: 10 in]
        n99 = Select(t=w296, s="Individual Plot Titles", f="ManualPlotTitles") -> (s? t:f=w294:string[])
        n100 = for {
          shift-right: [w346] -> w299
          shift-left: "" -> [w344]
          tunnel: w291 -> [w347]
          tunnel: "Plotstyles" -> [w348]
          tunnel: w294 -> [w330] mode=indexing
          tunnel: w292 -> [w343] mode=indexing
          tunnel: w290 -> [w333] mode=indexing
          tunnel: w289 -> [w332]
          tunnel: "LegendProperties" -> [w329]
          tunnel: "Title Offset (characters)" -> [w327]
          tunnel: w285 -> [w326]
          tunnel: w283 -> [w325]
          tunnel: w281 -> [w324]
          tunnel: w280 -> [w323]
          tunnel: w279 -> [w322]
          tunnel: w277 -> [w321]
          tunnel: "Y/R tics And Grids" -> [w320]
          tunnel: "X/Theta tics And Grids" -> [w319]
          tunnel: "xAxisBounds" -> [w318]
          # "Loops once for each graph on the multiplot"
          n101 = Unbundle By Name(w343) -> ("title"=w342:bool, "key"=w340:bool, "Xtic"=w337:bool, "Xlab"=w336:bool, "Ytic"=w335:bool, "Ylab"=w334:bool)
          n102 = call "TypesetInsideMathmode.vi"("DirtyString"=w330) -> ("De-dollared String"=w331:string)  [unwired: 9 in, 1 out]
          n103 = call "BuildPlotsOneGraph.vi"("Legend"=w332, "Desired Legends"=w333, "Plot Legends"=w347, "Plotstyles"=w348, "PlotCommand"=w326) -> ("String out"=w345:string)  [unwired: 6 in]
          n104 = call "setTitle.vi"("Offset"=w327, "Set?"=w342, "Title"=w331, "String in"=w344) -> ("String out"=w341:string)  [unwired: 6 in, 1 out]
          n105 = call "setKey.vi"("LegendProperties"=w329, "Set?"=w340, "String in"=w341) -> ("String out"=w339:string)  [unwired: 7 in, 1 out]
          n106 = call "AxisControl.vi"("ticsAndGrids"=w319, "Axis Label"=w325, "AxisBounds"=w318, "ShowLabel?"=w336, "ShowNumbers?"=w337, "Axis"=w323, "String in"=w339) -> ("String out"=w328:string)  [unwired: 3 in, 1 out]
          n107 = call "AxisControl.vi"("ticsAndGrids"=w320, "Axis Label"=w321, "AxisBounds"=w324, "ShowLabel?"=w334, "ShowNumbers?"=w335, "Axis"=w322, "String in"=w328) -> ("String out"=w338:string)  [unwired: 3 in, 1 out]
          n108 = Concatenate Strings(w338, w345) -> (w346:string)
        }
        n109 = Concatenate Strings(w298, w299, "\nunset multiplot\n") -> (w304:string)
      }
      frame "Write gnuplot file" {
        w356 = FALSE  # append to file? (new file:F)
        w357 = FALSE  # advisory dialog? (display:T)
        n110 = Strip Path(path=w353) -> (stripped path=w350:path)  [unwired: 1 out]
        n111 = Build Path(base path=w350, name or relative path="gnuplot_script.txt") -> (appended path=w358:path)
        n112 = call "Write_Characters_To_File.vi"("file path (dialog if empty)"=w358, "advisory dialog? (display:T)"=w357, "character string"=w349, "append to file? (new file:F)"=w356) -> ()  [unwired: 1 in, 4 out]
      }
      frame "Execute shell script" {
        n113 = call "Run_Gnuplot_Script.vi"("logfileName"=w360, "workingDirectory"=w361) -> ()
      }
      frame "Has pdf been generated?" {
        n114 = Select(t="Open Standard output file" ("f"), s="OpenLogfile?", f="End") -> (s? t:f=w367:string)
        n115 = Select(t="Show Re-Run Gnuplot?", s="Show Script Editor?", f=w367) -> (s? t:f=w371:string)
      }
      frame "Show Re-Run Gnuplot?" {
        n116 = Strip Path(path=w380) -> (stripped path=w379:path)  [unwired: 1 out]
        n117 = call "Re_run_Gnuplot.vi"("Plot folder (dialog if empty)"=w379) -> ()  [unwired: 4 out]
      }
      frame "Open Standard output file" {
        n118 = Strip Path(path=w390) -> (stripped path=w387:path)  [unwired: 1 out]
        n119 = Format Into String(format string="open \"%s\"", w388) -> (resulting string=w386:string)  [unwired: 2 in, 1 out]
        n120 = call <vilib>:"System Exec.vi"("working directory"=w387, "command line"=w386) -> ()  [unwired: 4 in, 6 out]
      }
      frame "End" {
      }
    }
    "gnuplotScript" <- w15
  }
  "AuditTrail" <- w2
  "Saved Automatically?" <- FALSE
